vi "Main_rownolegle.vi"() -> ()   [LabVIEW 2013]
doc: "Use this template to build a producer/consumer design pattern. Use this template when you need to execute a process, such as data analysis, when a data source, such as a triggered acquisition, produces data at an uneven rate and you need to execute the process when the data becomes available."
uses:
  inne pliki/Params.ctl
  inne pliki/Stany.ctl
  inne pliki/Data.ctl
  inne pliki/Akcje rownolegle FVG.ctl
panel:
  out "Czas":string
  in  "Zakres uśredniania (5)":i32=5
  in  "Temp limits":T1={"Max (25)"=25.0, "Min (0)"=0.0}
  out "Waveform Chart":T2(graph)
  out "Warning text":string
  out "Warning":bool
  in  "stop":bool
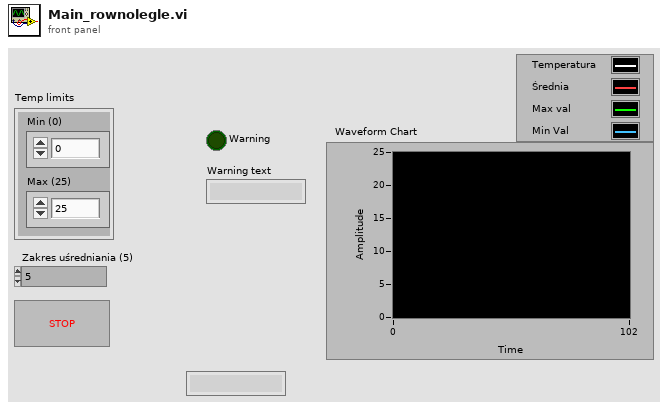
[diagram p1: front panel]
types:
  T1 = typedef "Params.ctl" = cluster{"Max (25)":dbl, "Min (0)":dbl}
  T2 = cluster{"Temperatura":dbl, "Średnia":dbl, "Max (25)":dbl, "Min (0)":dbl}
  T3 = enum16{"open", "replace", "create", "open or create", "replace or create", "replace or create with confirmation"}
  T4 = typedef "Data.ctl" = cluster{"Temperatura":dbl, "Średnia":dbl, "Warning":bool, "Warning text ":string, "Temp limits":T1, "Temp Array":dbl[], "Sternia Array":dbl[]}
  T5 = typedef "Stany.ctl" = enum16{"Config", "IDLE", "Measure", "Analyze", "Display", "STOP", "Save", "Error", "Error end"}
  T6 = typedef "Akcje rownolegle FVG.ctl" = enum16{"SET", "GET"}
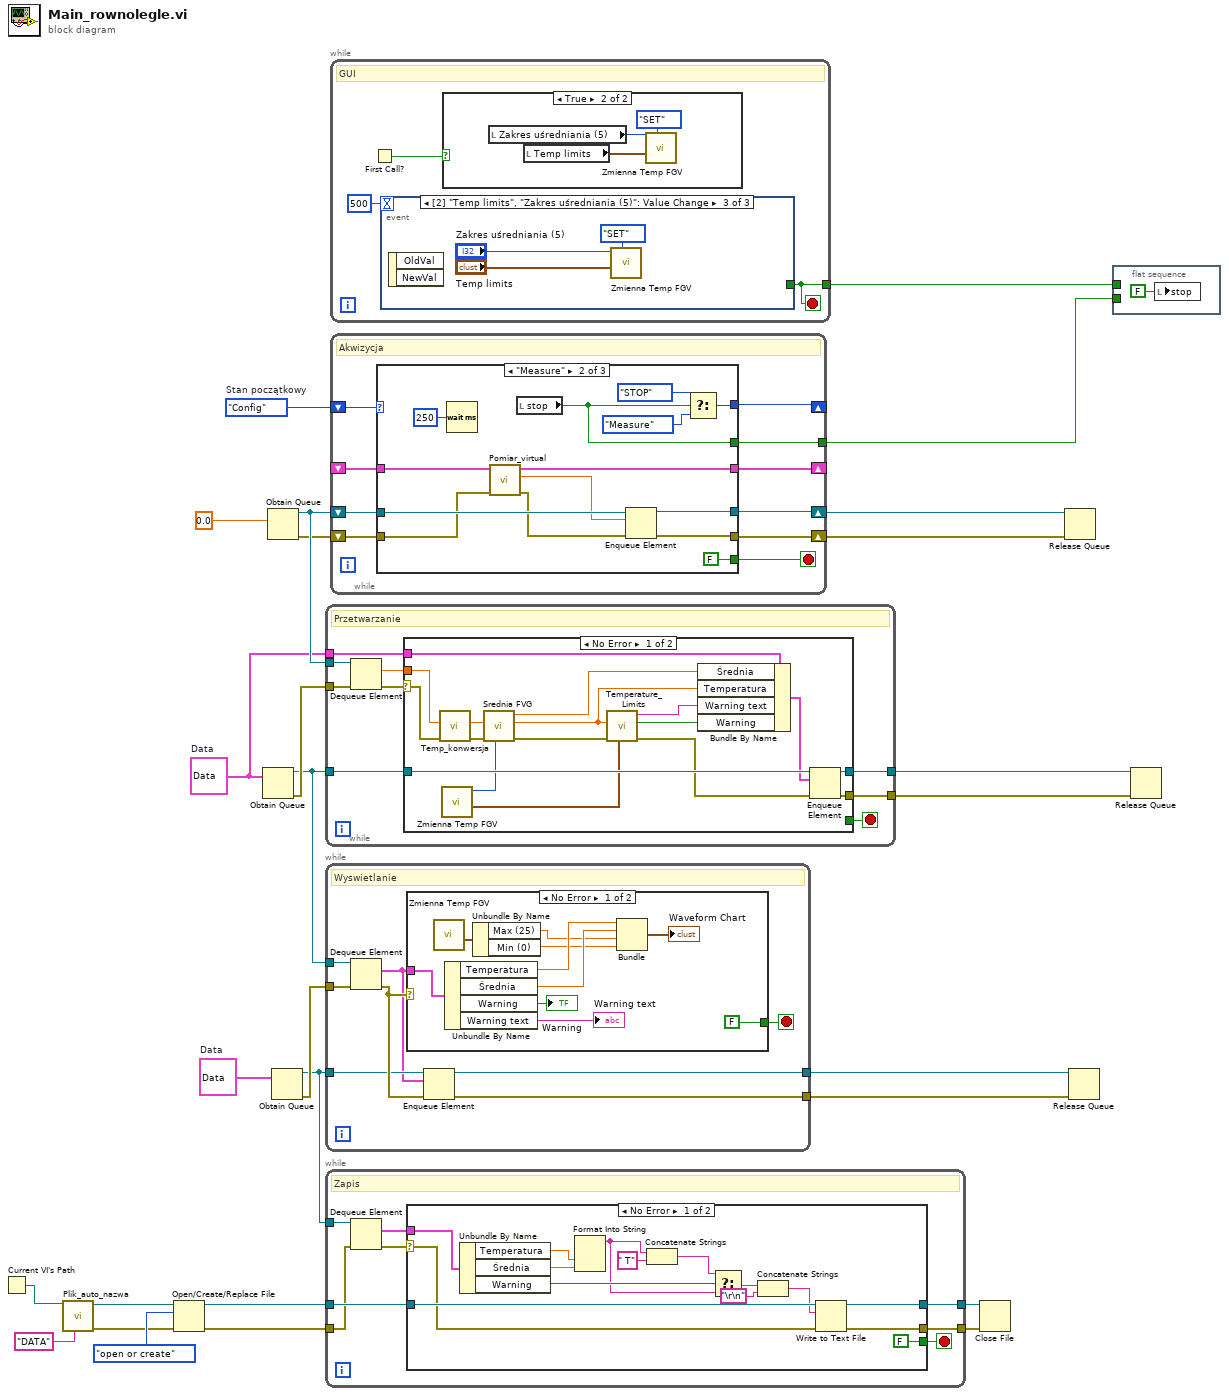
[diagram p0: block diagram]
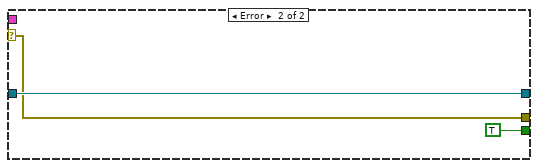
[diagram p2: hidden frame]
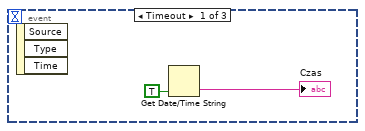
[diagram p4: hidden frame]
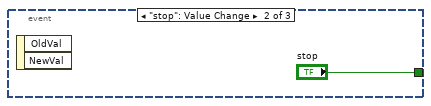
[diagram p5: hidden frame]
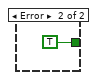
[diagram p6: hidden frame]
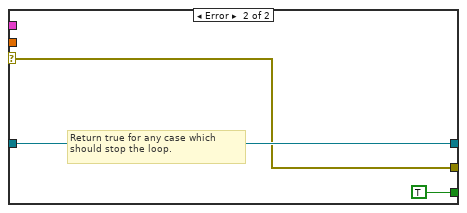
[diagram p7: hidden frame]
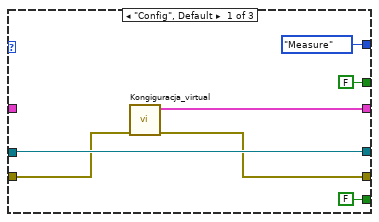
[diagram p8: hidden frame]
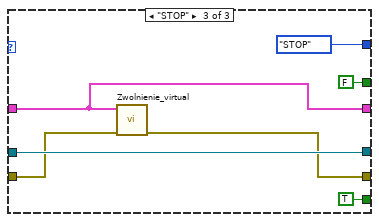
[diagram p9: hidden frame]
diagram:
  w14 = T4 {"Temperatura"=0.0, "Średnia"=0.0, "Warning"=FALSE, "Warning text "="", "Temp limits"={"Max (25)"=25.0, "Min (0)"=0.0}, "Temp Array"=[], "Sternia Array"=[]}  # Data
  w17 = T4 {"Temperatura"=0.0, "Średnia"=0.0, "Warning"=FALSE, "Warning text "="", "Temp limits"={"Max (25)"=25.0, "Min (0)"=0.0}, "Temp Array"=[], "Sternia Array"=[]}  # Data
  w23 = Stany."Config"  # Stan początkowy
  n1 = Current VI's Path() -> (path=w2:path)
  n2 = call "Plik_auto_nazwa.vi"("Nazwa in"="DATA", "path in"=w2) -> ("error out"=w1:errorcluster, "path out"=w5:path)  [unwired: 8 in]
  n3 = Open/Create/Replace File(file path (use dialog)=w5, error in=w1, operation (0:open)=T3."open or create") -> (refnum out=w9:refnum<file>, error out=w8:errorcluster)  [unwired: 3 in, 1 out]
  n4 = Obtain Queue(element data type=w17) -> (queue out=w18:refnum<queue>, error out=w21:errorcluster)  [unwired: 4 in, 1 out]
  n5 = Obtain Queue(element data type=0.0) -> (queue out=w27:refnum<queue>, error out=w26:errorcluster)  [unwired: 4 in, 1 out]
  n6 = Obtain Queue(element data type=w14) -> (queue out=w10:refnum<queue>, error out=w13:errorcluster)  [unwired: 4 in, 1 out]
  n7 = while {
    tunnel: w27 -> [w36]
    tunnel: w18 -> [w32]
    tunnel: w21 -> [w31]
    tunnel: [w30] -> w20
    tunnel: [w29] -> w19
    tunnel: w17 -> [w28]
    stop <- w33 stop-if-true
    # "Przetwarzanie"
    n8 = Dequeue Element(queue=w36, error in (no error)=w31) -> (element=w34:dbl, error out=w35:errorcluster)  [unwired: 1 in, 2 out]
    n9 = case shown="No Error" w35 {
      selector: w35 -> [w50 w54]
      tunnel: w34 -> [w51 _]
      tunnel: [_ TRUE] -> w33
      tunnel: w32 -> [w49 w55]
      tunnel: [w46 w55] -> w30
      tunnel: [w45 w54] -> w29
      tunnel: w28 -> [w39 _]
      frame No Error {
        n10 = call "Temp_konwersja.vi"("error in (no error)"=w50, "Temp in"=w51) -> ("error out"=w52:errorcluster, "Temp out"=w53:dbl)  [unwired: 8 in]
        n11 = call "Zmienna Temp FGV.vi"() -> ("Temp limits out"=w37:T1, "Zakres out"=w38:i32)  [unwired: 9 in, 1 out]
        n12 = call "Srednia FVG.vi"("Zakres (5)"=w38, "error in (no error)"=w52, "temperatura in"=w53) -> ("error out"=w48:errorcluster, "temperatura out"=w43:dbl, "średnia out"=w44:dbl)  [unwired: 6 in]
        n13 = call "Temperature_Limits.vi"("Temp limits"=w37, "error in (no error)"=w48, "TEMP"=w43) -> ("error out"=w47:errorcluster, "Warning"=w41:bool, "Warning Text"=w42:string)  [unwired: 6 in]
        n14 = Bundle By Name(cluster=w39, "Średnia"=w44, "Temperatura"=w43, "Warning text"=w42, "Warning"=w41) -> (w40:T4)
        n15 = Enqueue Element(queue=w49, element=w40, error in (no error)=w47) -> (queue out=w46:refnum<queue>, error out=w45:errorcluster)  [unwired: 1 in, 1 out]
      }
      frame Error {
        # "Return true for any case which should stop the loop."
      }
    }
  }
  n16 = while {
    tunnel: w18 -> [w64]
    tunnel: w13 -> [w62]
    tunnel: w10 -> [w60]
    tunnel: [w58] -> w12
    tunnel: [w57] -> w11
    stop <- w63 stop-if-true
    # "Wyswietlanie"
    n17 = Dequeue Element(queue=w64, error in (no error)=w62) -> (element=w59:T4, error out=w61:errorcluster)  [unwired: 1 in, 2 out]
    n18 = case shown="No Error" w61 {
      tunnel: w59 -> [w74 _]
      tunnel: [FALSE TRUE] -> w63
      frame No Error {
        n19 = call "Zmienna Temp FGV.vi"() -> ("Temp limits out"=w67:T1)  [unwired: 9 in, 2 out]
        n20 = Unbundle By Name(w74) -> ("Temperatura"=w70:dbl, "Średnia"=w69:dbl, "Warning"=→"Warning":bool, "Warning text"=→"Warning text":string)
        n21 = Unbundle By Name(w67) -> ("Max (25)"=w66:dbl, "Min (0)"=w65:dbl)
        n22 = Bundle("Temperatura"=w70, "Średnia"=w69, "Max (25)"=w66, "Min (0)"=w65) -> (→"Waveform Chart":T2)  [unwired: 1 in]
      }
      frame Error {
      }
    }
    n23 = Enqueue Element(queue=w60, element=w59, error in (no error)=w61) -> (queue out=w58:refnum<queue>, error out=w57:errorcluster)  [unwired: 1 in, 1 out]
  }
  n24 = while {
    tunnel: w10 -> [w83]
    tunnel: w9 -> [w79]
    tunnel: w8 -> [w78]
    tunnel: [w77] -> w7
    tunnel: [w76] -> w6
    stop <- w82 stop-if-true
    # "Zapis"
    n25 = Dequeue Element(queue=w83, error in (no error)=w78) -> (element=w80:T4, error out=w81:errorcluster)  [unwired: 1 in, 2 out]
    n26 = case shown="No Error" w81 {
      selector: w81 -> [w96 w99]
      tunnel: w80 -> [w93 _]
      tunnel: [FALSE TRUE] -> w82
      tunnel: w79 -> [w97 w100]
      tunnel: [w95 w99] -> w77
      tunnel: [w94 w100] -> w76
      frame No Error {
        n27 = Unbundle By Name(w93) -> ("Temperatura"=w92:dbl, "Średnia"=w91:dbl, "Warning"=w89:bool)
        n28 = Format Into String "Format Into String"(w92, w91) -> (resulting string=w87:string)  [unwired: 3 in, 1 out]
        n29 = Concatenate Strings(w87, " T" ("string")) -> (w88:string)
        n30 = Select(t=w88, s=w89, f=w87) -> (s? t:f=w86:string)
        n31 = Concatenate Strings(w86, "\r\n") -> (w85:string)
        n32 = Write to Text File(file (use dialog)=w97, text=w85, error in=w96) -> (refnum out=w94:refnum<file>, error out=w95:errorcluster)  [unwired: 1 in, 1 out]
      }
      frame Error {
      }
    }
  }
  n33 = while {
    tunnel: [w104] -> w16
    stop <- w104 stop-if-true
    # "GUI"
    n34 = First Call?() -> (First Call?: T/F=w103:bool)
    n35 = event shown="[2] \"Temp limits\", \"Zakres uśredniania (5)\": Value Change" {
      selector: _ -> [_ _ _]
      dyn-events: _ -> [_ _ _]
      timeout: 500 -> [_ _ _]
      tunnel: [_ "stop" _] -> w104
      event Timeout {
        n36 = event-data() -> ()  [unwired: 1 in, 3 out]
        n37 = Get Date/Time String(want seconds? (F)=TRUE) -> (time string=→"Czas":string)  [unwired: 2 in, 1 out]
      }
      event "stop": Value Change {
        n38 = event-data() -> ()  [unwired: 1 in, 2 out]
      }
      event "Zakres uśredniania (5)": Value Change {
        n39 = event-data() -> ()  [unwired: 1 in, 2 out]
        n40 = call "Zmienna Temp FGV.vi"("Akcje (GET)"=Akcje_rownolegle_FVG."SET", "Temp limits in"="Temp limits", "Zakres in"="Zakres uśredniania (5)") -> ()  [unwired: 6 in, 3 out]
      }
    }
    n41 = case shown="True" w103 {
      frame False {
      }
      frame True {
        n42 = local read "Zakres uśredniania (5)"() -> (w105:i32)
        n43 = local read "Temp limits"() -> (w106:T1)
        n44 = call "Zmienna Temp FGV.vi"("Akcje (GET)"=Akcje_rownolegle_FVG."SET", "Temp limits in"=w106, "Zakres in"=w105) -> ()  [unwired: 6 in, 3 out]
      }
    }
  }
  n45 = while {
    shift-right: [w118] -> w24
    shift-left: w26 -> [w117]
    shift-right: [w119] -> w25
    shift-left: w27 -> [w120]
    shift-right: [w122] -> _
    shift-left: w23 -> [w123]
    shift-right: [w116] -> _
    shift-left: _ -> [w115]
    tunnel: [w114] -> w15
    stop <- w121 stop-if-true
    # "Akwizycja"
    n46 = case shown="\"Measure\"" w123 {
      tunnel: [Stany."Measure" ("Stan") w142 Stany."STOP" ("Stan")] -> w122
      tunnel: [FALSE FALSE TRUE] -> w121
      tunnel: w120 -> [w128 w140 w149]
      tunnel: [w128 w139 w149] -> w119
      tunnel: [w125 w135 w147] -> w118
      tunnel: w117 -> [w126 w133 w148]
      tunnel: [w127 w137 w146] -> w116
      tunnel: w115 -> [_ w138 w146]
      tunnel: [FALSE ("stop") w131 FALSE ("stop")] -> w114
      frame "Config", Default {
        n47 = call "Kongiguracja_virtual.vi"("error in (no error)"=w126) -> ("error out"=w125:errorcluster, "Reference out"=w127:cluster{"Numeric":dbl, "Boolean":bool})  [unwired: 9 in]
      }
      frame "Measure" {
        n48 = Wait (ms)(milliseconds to wait=u32 250) -> ()  [unwired: 1 out]
        n49 = call "Pomiar_virtual.vi"("error in (no error)"=w133, "Reference in"=w138) -> ("error out"=w134:errorcluster, "out"=w136:dbl, "Reference out"=w137:cluster{"Numeric":dbl, "Boolean":bool})  [unwired: 7 in]
        n50 = local read "stop"() -> (w131:bool)
        n51 = Enqueue Element(queue=w140, element=w136, error in (no error)=w134) -> (queue out=w139:refnum<queue>, error out=w135:errorcluster)  [unwired: 1 in, 1 out]
        n52 = Select(t=Stany."STOP" ("Stan"), s=w131, f=Stany."Measure" ("Stan")) -> (s? t:f=w142:T5)
      }
      frame "STOP" {
        n53 = call "Zwolnienie_virtual.vi"("error in (no error)"=w148, "Reference in"=w146) -> ("error out"=w147:errorcluster)  [unwired: 9 in]
      }
    }
  }
  n54 = Close File(refnum=w6, error in=w7) -> ()  [unwired: 2 out]
  n55 = Release Queue(queue=w25, error in (no error)=w24) -> ()  [unwired: 1 in, 3 out]
  n56 = Release Queue(queue=w12, error in (no error)=w11) -> ()  [unwired: 1 in, 3 out]
  n57 = flat-sequence {
    tunnel: w16 -> [_]
    tunnel: w15 -> [_]
    frame #0 {
      n58 = local write "stop"(FALSE ("stop")) -> ()
    }
  }
  n59 = Release Queue(queue=w20, error in (no error)=w19) -> ()  [unwired: 1 in, 3 out]
